vi "Write Exception Status.vi"(8 "error in (no error)":errorcluster, 10 "exception status":u8 format="%02x", 11 "MB CR in":refnum<class "Modbus Master CR API.lvclass">) -> (0 "error out":errorcluster, 3 "MB CR out":refnum<class "Modbus Master CR API.lvclass">)   [LabVIEW 2021, in "Modbus Master CR API.lvclass"]
doc: "Writes the exception status of a Modbus slave. The exception status is a set of eight status bits. Each status bit represents an exception."
uses:
  Modbus Master CR API.lvclass
  D:/my_projects/projects/Algorithms/Labview/21/Modbus_v121c/API/Modbus API.lvclass
  Modbus API.lvclass/Modbus API.ctl
  Network Protocol/MB/Modbus Master CR.lvclass/Modbus Master CR.ctl
  Read Network Protocol.vi
  Network Protocol/MB/Modbus Master CR.lvclass
  Data Model/Device Data Model.lvclass
  Modbus Master CR API.lvclass/Modbus Master CR API.ctl
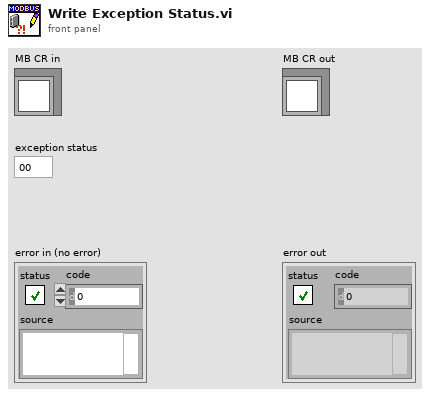
[diagram p1: front panel]
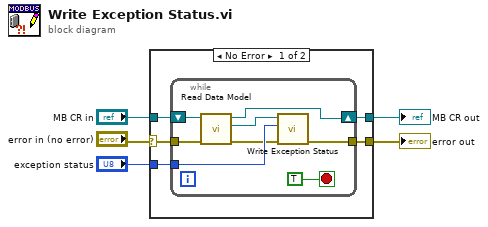
[diagram p0: block diagram]
diagram:
  n1 = case shown="No Error" "error in (no error)" {
    selector: "error in (no error)" -> [w8 w19]
    tunnel: "MB CR in" -> [w10 w20]
    tunnel: [w9 w20] -> w4
    tunnel: [w7 w19] -> w2
    tunnel: "exception status" -> [w6 _]
    frame No Error {
      n2 = while {
        shift-right: [w12] -> w9
        shift-left: w10 -> [w11]
        tunnel: w8 -> [w15]
        tunnel: [w18] -> w7
        tunnel: w6 -> [w17]
        stop <- TRUE stop-if-true
        n3 = call "Read Data Model.vi"("error in (no error)"=w15, "MB CR in"=w11) -> ("error out"=w14:errorcluster, "device data model"=w13:refnum<class "Device Data Model.lvclass">, "MB CR out"=w12:refnum<class "Modbus Master CR API.lvclass">)  [unwired: 7 in]
        n4 = call-dynamic "Write Exception Status.vi"("error in"=w14, "exception status"=w17, "device data model in"=w13) -> ("error out"=w18:errorcluster)  [unwired: 7 in, 1 out]
      }
    }
    frame Error {
    }
  }
  "MB CR out" <- w4
  "error out" <- w2
